vi "Rig_Pict_Display_Pref.vi"(0 "Traverse Name":string) -> (1 "Roll Pitch Yaw ADAM Channels":string[](array[string]), 4 "Which Axis is vertical?":enum16{"X Axis", "Y Axis", "Z Axis"}(ring), 6 "Plan View":T1, 7 "Side View":T1, 8 "Front View":T1)   [LabVIEW 2016]
uses:
  Pict_Plot_Axis.ctl
  Axis.ctl
  Globals/Constants_global.vi
  Globals/Trav_pos_global.vi
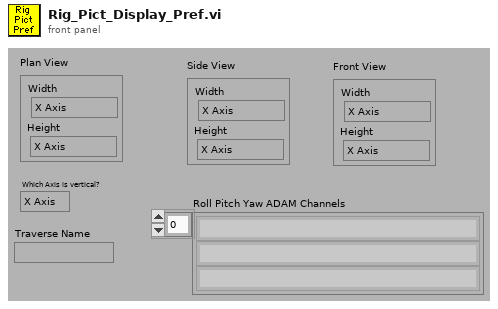
[diagram p1: front panel]
types:
  T1 = typedef "Pict_Plot_Axis.ctl" = cluster{"Width":T2, "Height":T2}
  T2 = typedef "Axis.ctl" = enum16{"X Axis", "X Axis -ve", "Y Axis", "Y Axis -ve", "Z Axis", "Z Axis -ve"}
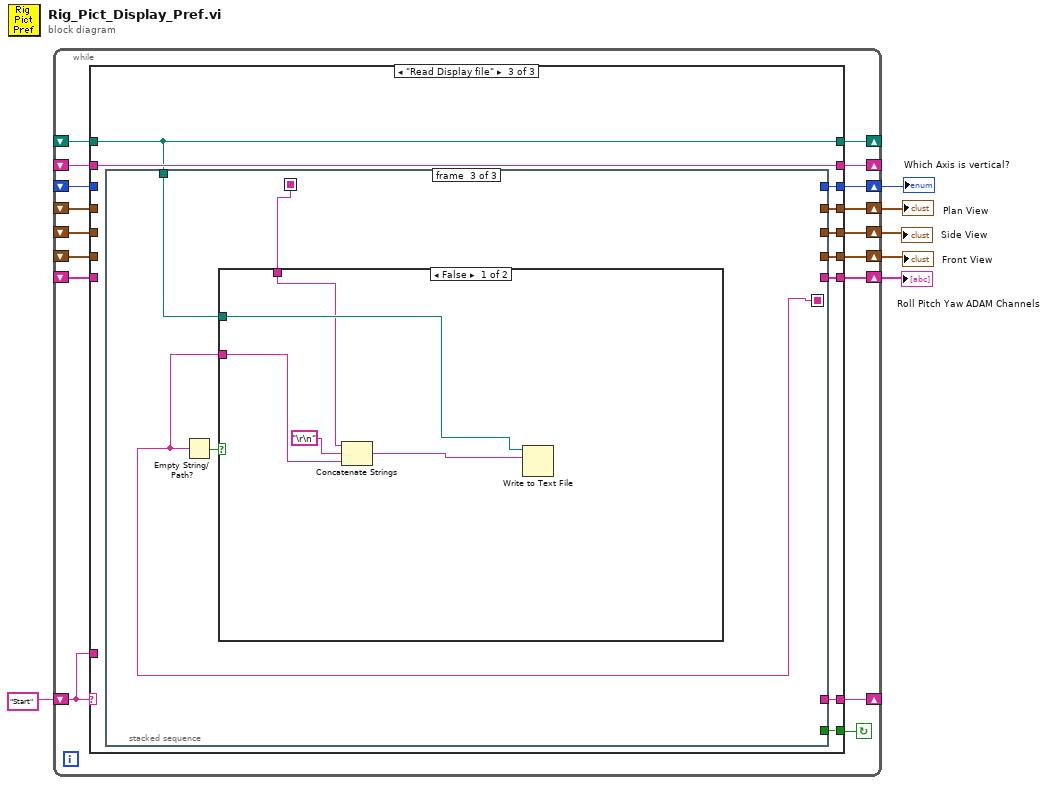
[diagram p0: block diagram]
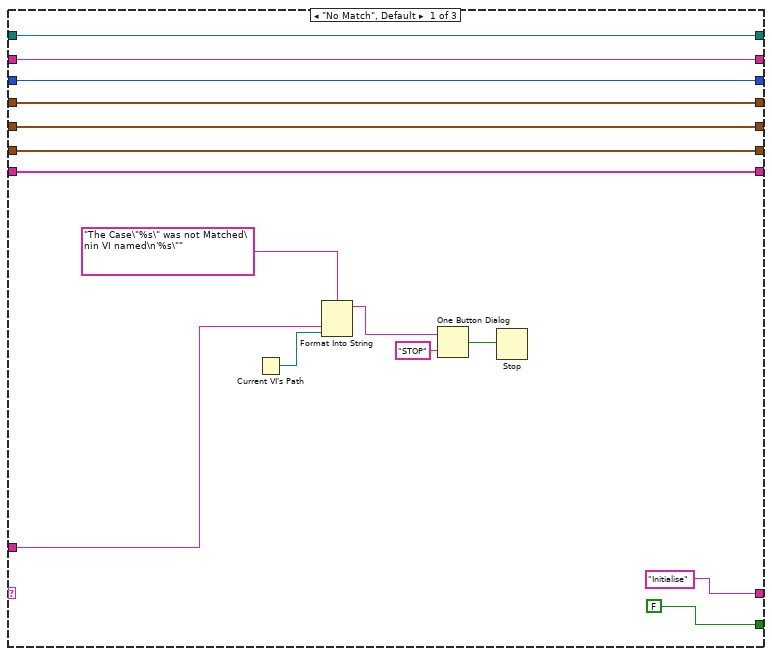
[diagram p2: hidden frame]
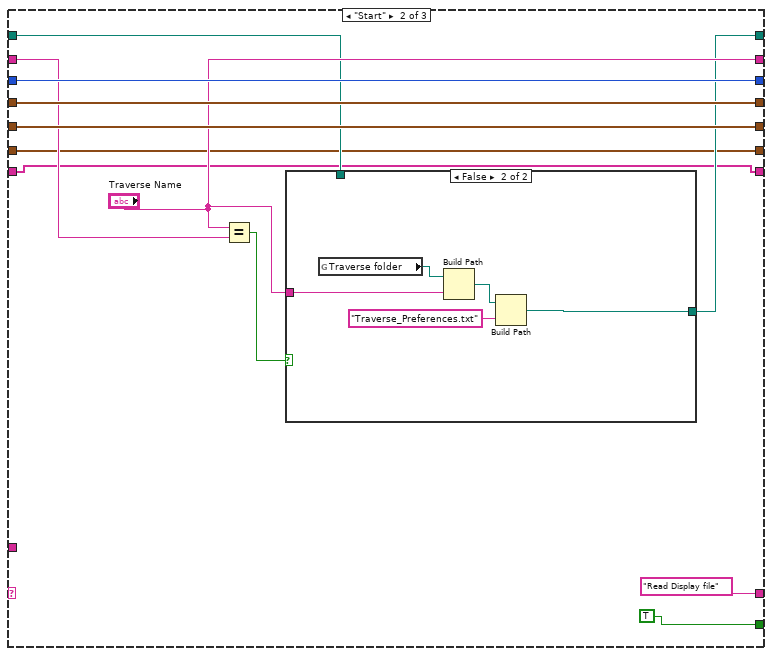
[diagram p3: hidden frame]
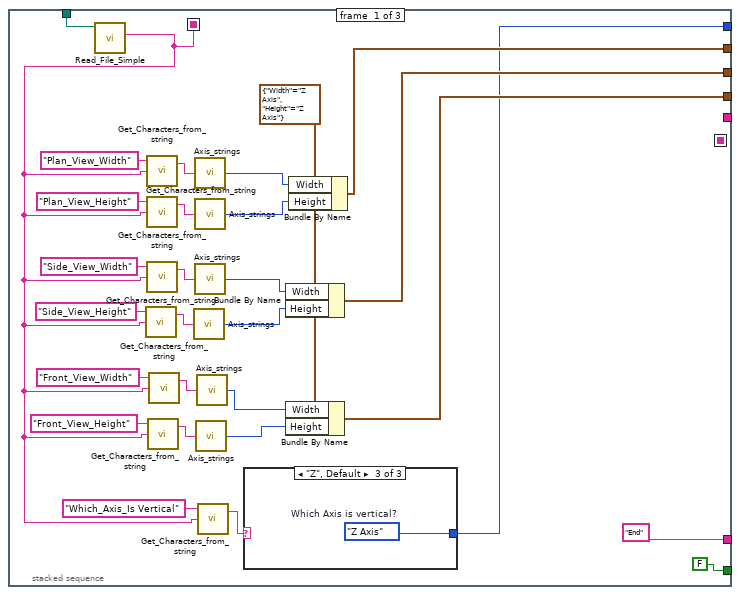
[diagram p5: hidden frame]
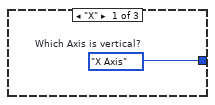
[diagram p6: hidden frame]
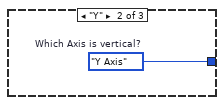
[diagram p7: hidden frame]
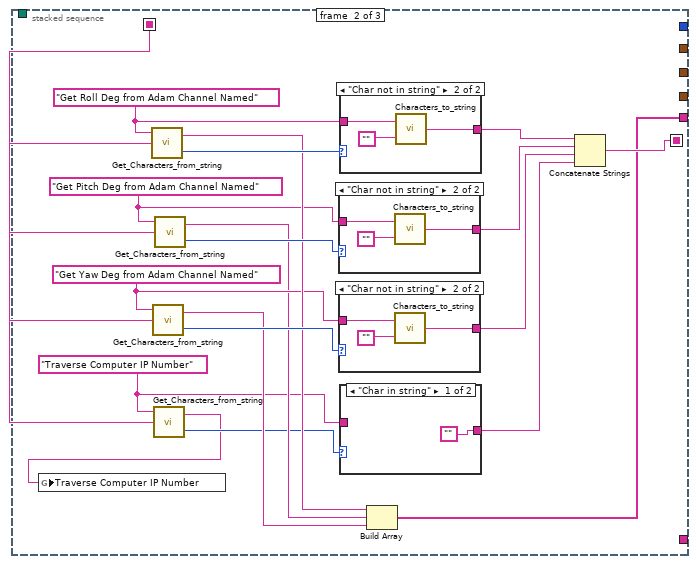
[diagram p8: hidden frame]
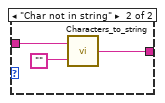
[diagram p9: hidden frame]
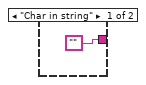
[diagram p10: hidden frame]
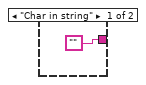
[diagram p11: hidden frame]
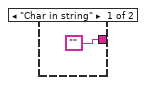
[diagram p12: hidden frame]
diagram:
  n1 = while {
    shift-left: "Start" -> [w21]
    shift-right: [w22] -> _
    shift-right: [w19] -> _
    shift-left: _ -> [w20]
    shift-right: [w13] -> w2
    shift-left: _ -> [w14]
    shift-right: [w16] -> w5
    shift-left: _ -> [w15]
    shift-right: [w17] -> w4
    shift-left: _ -> [w18]
    shift-right: [w12] -> _
    shift-left: _ -> [w11]
    shift-right: [w9] -> w3
    shift-left: _ -> [w10]
    shift-right: [w8] -> w1
    shift-left: _ -> [w7]
    stop <- w23 continue-if-true
    n2 = case shown="\"Read Display file\"" w21 {
      tunnel: [FALSE TRUE ("Modified?") w58] -> w23
      tunnel: ["Initialise" "Read Display file" w65] -> w22
      tunnel: w21 -> [w33 _ _]
      tunnel: w20 -> [w29 w46 w64]
      tunnel: [w29 "Traverse Name" w64] -> w19
      tunnel: w18 -> [w26 w49 _]
      tunnel: [w26 w49 w61] -> w17
      tunnel: [w27 w48 w62] -> w16
      tunnel: w15 -> [w27 w48 _]
      tunnel: w14 -> [w28 w47 _]
      tunnel: [w28 w47 w59] -> w13
      tunnel: [w30 w44 w63] -> w12
      tunnel: w11 -> [w30 w42 w63]
      tunnel: w10 -> [w25 w41 _]
      tunnel: [w25 w41 w60] -> w9
      tunnel: [w24 w40 w57] -> w8
      tunnel: w7 -> [w24 w40 _]
      frame "No Match", Default {
        n3 = Current VI's Path() -> (path=w32:path)
        n4 = Format Into String(format string="The Case\"%s\" was not Matched\nin VI named\n'%s\"" ("Format String"), w33, w32) -> (resulting string=w36:string)  [unwired: 2 in, 1 out]
        n5 = One Button Dialog(message=w36, button name ("OK")="STOP") -> (true=w34:bool)
        n6 = Stop(stop? (T)=w34) -> ()
      }
      frame "Start" {
        n7 = Equal?(x="Traverse Name", y=w46) -> (x = y?=w43:bool)
        n8 = case shown="False" w43 {
          tunnel: "Traverse Name" -> [_ w55]
          tunnel: [w51 w52] -> w44
          tunnel: w42 -> [w51 _]
          frame True {
          }
          frame False {
            n9 = global read "Constants_global.vi" "Traverse folder"() -> (w56:path)
            n10 = Build Path(base path=w56, name or relative path=w55) -> (appended path=w54:path)
            n11 = Build Path(base path=w54, name or relative path="Traverse_Preferences.txt") -> (appended path=w52:path)
          }
        }
      }
      frame "Read Display file" {
        n12 = stacked-sequence {
          seq-local: [w66 _ _] -> [_ w101 w135]
          seq-local: [_ w104 _] -> [_ _ w134]
          tunnel: ["End" _ _] -> w65
          tunnel: w63 -> [w93 _ w133]
          tunnel: [w73 _ _] -> w62
          tunnel: [w72 _ _] -> w61
          tunnel: [w71 _ _] -> w60
          tunnel: [w68 _ _] -> w59
          tunnel: [FALSE ("Modified?") _ _] -> w58
          tunnel: [_ w103 _] -> w57
          frame #0 {
            w78 = T1 {"Width"=enum."Z Axis", "Height"=enum."Z Axis"} ("Plot Axis")
            n13 = call "Read_File_Simple.vi"("Filename"=w93) -> ("string"=w66:string)  [unwired: 2 in, 7 out]
            n14 = call "Get_Characters_from_string.vi"("Input string"=w66, "Variable name"="Side_View_Height") -> ("Value"=w86:string)  [unwired: 1 in, 1 out]
            n15 = call "Get_Characters_from_string.vi"("Input string"=w66, "Variable name"="Plan_View_Width") -> ("Value"=w91:string)  [unwired: 1 in, 1 out]
            n16 = call "Get_Characters_from_string.vi"("Input string"=w66, "Variable name"="Plan_View_Height") -> ("Value"=w90:string)  [unwired: 1 in, 1 out]
            n17 = call "Get_Characters_from_string.vi"("Input string"=w66, "Variable name"="Side_View_Width") -> ("Value"=w87:string)  [unwired: 1 in, 1 out]
            n18 = call "Get_Characters_from_string.vi"("Input string"=w66, "Variable name"="Front_View_Height") -> ("Value"=w82:string)  [unwired: 1 in, 1 out]
            n19 = call "Get_Characters_from_string.vi"("Input string"=w66, "Variable name"="Front_View_Width") -> ("Value"=w83:string)  [unwired: 1 in, 1 out]
            n20 = call "Axis_strings.vi"("String"=w86) -> ("Enum"=w74:T2)
            n21 = call "Axis_strings.vi"("String"=w91) -> ("Enum"=w77:T2)
            n22 = call "Axis_strings.vi"("String"=w90) -> ("Enum"=w76:T2)
            n23 = call "Axis_strings.vi"("String"=w87) -> ("Enum"=w75:T2)
            n24 = call "Axis_strings.vi"("String"=w82) -> ("Enum"=w79:T2)
            n25 = call "Axis_strings.vi"("String"=w83) -> ("Enum"=w80:T2)
            n26 = call "Get_Characters_from_string.vi"("Input string"=w66, "Variable name"="Which_Axis_Is Vertical") -> ("Value"=w69:string)  [unwired: 1 in, 1 out]
            n27 = case shown="\"Z\", Default" w69 {
              tunnel: [w95 w96 w97] -> w68
              frame "X" {
                w95 = enum16{"X Axis", "Y Axis", "Z Axis"}."X Axis"  # Which Axis is vertical?
              }
              frame "Y" {
                w96 = enum16{"X Axis", "Y Axis", "Z Axis"}."Y Axis"  # Which Axis is vertical?
              }
              frame "Z", Default {
                w97 = enum16{"X Axis", "Y Axis", "Z Axis"}."Z Axis"  # Which Axis is vertical?
              }
            }
            n28 = Bundle By Name(cluster=w78, "Width"=w75, "Height"=w74) -> (w72:T1)
            n29 = Bundle By Name(cluster=w78, "Width"=w80, "Height"=w79) -> (w71:T1)
            n30 = Bundle By Name(cluster=w78, "Width"=w77, "Height"=w76) -> (w73:T1)
          }
          frame #1 {
            w100 = "Traverse Computer IP Number" ("Variable name")
            w107 = "Get Yaw Deg from Adam Channel Named" ("Variable name")
            w108 = "Get Pitch Deg from Adam Channel Named" ("Variable name")
            w115 = "Get Roll Deg from Adam Channel Named" ("Variable name")
            n31 = call "Get_Characters_from_string.vi"("Input string"=w101, "Variable name"=w115) -> ("Status"=w116:enum16{"Char in string", "Char not in string"}, "Value"=w109:string)  [unwired: 1 in]
            n32 = call "Get_Characters_from_string.vi"("Input string"=w101, "Variable name"=w107) -> ("Status"=w112:enum16{"Char in string", "Char not in string"}, "Value"=w105:string)  [unwired: 1 in]
            n33 = call "Get_Characters_from_string.vi"("Input string"=w101, "Variable name"=w100) -> ("Status"=w102:enum16{"Char in string", "Char not in string"}, "Value"=w98:string)  [unwired: 1 in]
            n34 = global write "Trav_pos_global.vi" "Traverse Computer IP Number"(w98) -> ()
            n35 = call "Get_Characters_from_string.vi"("Input string"=w101, "Variable name"=w108) -> ("Status"=w113:enum16{"Char in string", "Char not in string"}, "Value"=w106:string)  [unwired: 1 in]
            n36 = case shown="\"Char not in string\"" w113 {
              tunnel: w108 -> [_ w128]
              tunnel: ["" w126] -> w111
              frame "Char in string" {
              }
              frame "Char not in string" {
                n37 = call "Characters_to_string.vi"("Characters to write"="", "Label for characters"=w128) -> ("Output string"=w126:string)
              }
            }
            n38 = case shown="\"Char not in string\"" w112 {
              tunnel: w107 -> [_ w124]
              tunnel: ["" w122] -> w110
              frame "Char in string" {
              }
              frame "Char not in string" {
                n39 = call "Characters_to_string.vi"("Characters to write"="", "Label for characters"=w124) -> ("Output string"=w122:string)
              }
            }
            n40 = case shown="\"Char not in string\"" w116 {
              tunnel: w115 -> [_ w132]
              tunnel: ["" w130] -> w114
              frame "Char in string" {
              }
              frame "Char not in string" {
                n41 = call "Characters_to_string.vi"("Characters to write"="", "Label for characters"=w132) -> ("Output string"=w130:string)
              }
            }
            n42 = case shown="\"Char in string\"" w102 {
              tunnel: w100 -> [_ w120]
              tunnel: ["" w118] -> w99
              frame "Char in string" {
              }
              frame "Char not in string" {
                n43 = call "Characters_to_string.vi"("Characters to write"="", "Label for characters"=w120) -> ("Output string"=w118:string)
              }
            }
            n44 = Build Array(w109, w106, w105) -> (w103:string[])
            n45 = Concatenate Strings(w114, w111, w110, w99) -> (w104:string)
          }
          frame #2 {
            n46 = Empty String/Path?(string/path=w134) -> (empty?=w136:bool)
            n47 = case shown="False" w136 {
              tunnel: w135 -> [w137 _]
              tunnel: w134 -> [w140 _]
              tunnel: w133 -> [w139 _]
              frame False {
                n48 = Concatenate Strings(w137, "\r\n", w140) -> (w138:string)
                n49 = Write to Text File(file (use dialog)=w139, text=w138) -> ()  [unwired: 2 in, 3 out]
              }
              frame True {
              }
            }
          }
        }
      }
    }
  }
  "Plan View" <- w5
  "Side View" <- w4
  "Front View" <- w3
  "Which Axis is vertical?" <- w2
  "Roll Pitch Yaw ADAM Channels" <- w1
